vi "createMotionProfile.vi"(6 "ms per frame":dbl=50.0, 8 "Max Jerk (In/sec^3)":dbl=60.0, 9 "Max Acceleration (In/sec^2)":dbl=80.0, 10 "Max Speed (In/sec)":dbl=120.0, 11 "Inches to Travel":dbl=250.0) -> (3 "Profile":cluster{"Pos":dbl[], "Vel":dbl[], "accel":dbl[]})   [LabVIEW 2016]
panel:
  out "Final Position":dbl
  out "XY Graph":cluster{dbl[], dbl[]}[](graph)
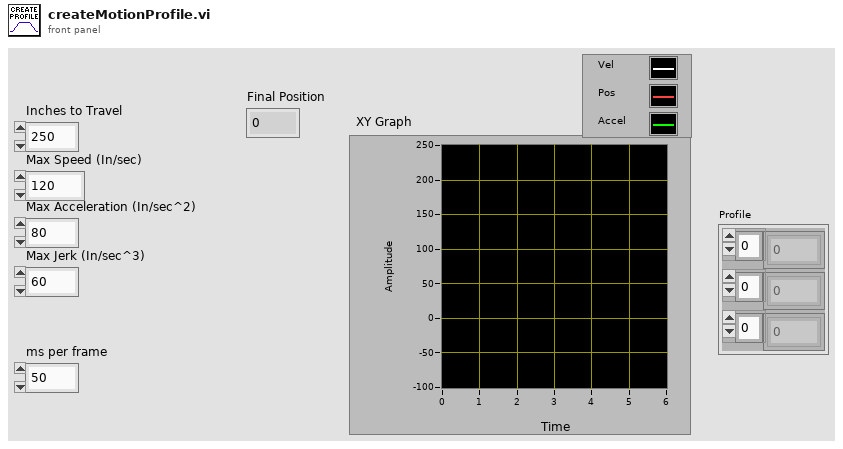
[diagram p1: front panel]
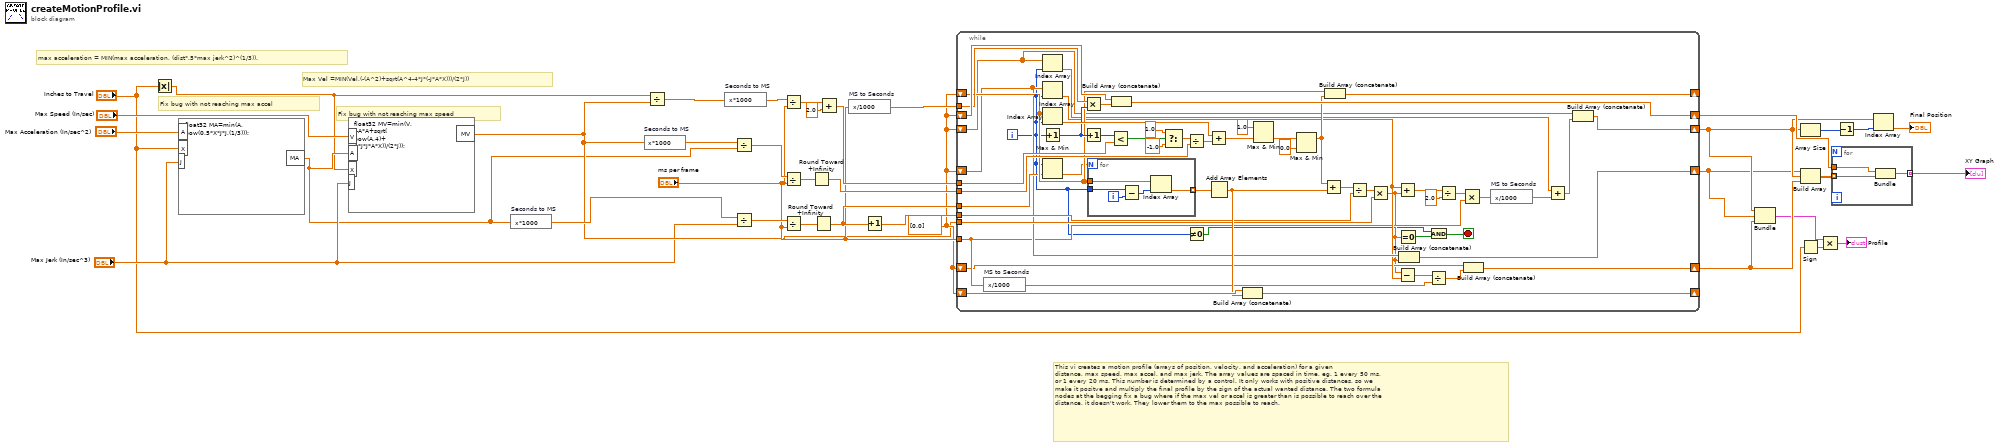
[diagram p0: block diagram]
diagram:
  w20 = dbl[] [0.0]
  # "Fix bug with not reaching max accel"
  # "max acceleration = MIN(max acceleration, (dist*.5*max jerk^2)^(1/3))."
  # "This vi creates a motion profile (arrays of position, velocity, and acceleration) for a given\ndistance, max speed, max accel, and max jerk. The array values are spaced in time, eg. 1 every 50 ms, \nor 1 every 20 ms. This number is determined by a control. It only works with positive distances, so we \nmake it positve and multiply the final profile by the sign of the actual wanted distance. The two formula\nnodes at the begging fix a bug where if the max vel or accel is greater than is possible to reach over the\ndistance, it doesn't work. They lower them to the max possible to reach."
  # "Fix bug with not reaching max speed"
  # "Max Vel =MIN(Vel,(-(A^2)+sqrt(A^4-4*J*(-J*A*X)))/(2*J))"
  n1 = Absolute Value(x="Inches to Travel") -> (abs(x)=w1:dbl)
  n2 = formula code="float32 MA=min(A,\npow(0.5*X*J*J,(1/3)));"("A"="Max Acceleration (In/sec^2)", "X"="Inches to Travel", "J"="Max Jerk (In/sec^3)") -> ("MA"=w9:sgl)
  n3 = formula code="float32 MV=min(V,\n(-A*A+sqrt(\npow(A,4)+\n4*J*J*A*X))/(2*J));"("V"="Max Speed (In/sec)", "A"=w9, "X"=w1, "J"="Max Jerk (In/sec^3)") -> ("MV"=w13:sgl)
  n4 = expression code="x*1000" "Seconds to MS"(w9) -> (w35:sgl)
  n5 = expression code="x*1000" "Seconds to MS"(w13) -> (w34:sgl)
  n6 = Divide(x=w1, y=w13) -> (x/y=w33:dbl)
  n7 = expression code="x*1000" "Seconds to MS"(w33) -> (w32:dbl)
  n8 = Divide(x=w34, y=w9) -> (x/y=w28:sgl)
  n9 = Divide(x=w35, y="Max Jerk (In/sec^3)") -> (x/y=w25:dbl)
  n10 = Divide(x=w32, y="ms per frame") -> (x/y=w31:dbl)
  n11 = Divide(x=w28, y="ms per frame") -> (x/y=w27:dbl)
  n12 = Divide(x=w25, y="ms per frame") -> (x/y=w24:dbl)
  n13 = Round Toward +Infinity(x=w27) -> (ceil(x): smallest int >= x=w26:dbl)
  n14 = Round Toward +Infinity(x=w24) -> (ceil(x): smallest int >= x=w23:dbl)
  n15 = Add(x=w31, y=2.0) -> (x+y=w29:dbl)
  n16 = expression code="x/1000" "MS to Seconds"("ms per frame") -> (w36:dbl)
  n17 = Increment(x=w23) -> (x+1=w22:dbl)
  n18 = while {
    shift-right: [w89] -> w18
    shift-left: w20 -> [w90]
    tunnel: w36 -> [w88]
    tunnel: w29 -> [w86]
    shift-right: [w72] -> _
    shift-left: w20 -> [w71]
    tunnel: w26 -> [w78]
    tunnel: w23 -> [w69]
    shift-right: [w66] -> _
    shift-left: w20 -> [w67]
    tunnel: w22 -> [w62]
    tunnel: w13 -> [w60]
    shift-right: [w59] -> w6
    shift-left: w20 -> [w57]
    shift-right: [w58] -> w8
    shift-left: w20 -> [w51]
    tunnel: "ms per frame" -> [w45]
    shift-right: [w43] -> w7
    shift-left: w20 -> [w42]
    i -> [w41]
    stop <- w37 stop-if-true
    n19 = expression code="x/1000" "MS to Seconds"(w45) -> (w46:dbl)
    n20 = Index Array(array=w51, index=w41) -> (element=w50:dbl)
    n21 = Index Array(array=w57, index=w41) -> (element=w48:dbl)
    n22 = Index Array(array=w71, index=w41) -> (element=w76:dbl)
    n23 = Increment(x=w41) -> (x+1=w74:i32)
    n24 = Max & Min(x=w41, y=w69) -> (min(x,y)=w68:dbl)  [unwired: 1 out]
    n25 = Multiply(x=w88, y=w74) -> (x*y=w87:dbl)
    n26 = Increment(x=w74) -> (x+1=w75:i32)
    n27 = for {
      N: w68 -> [_]
      tunnel: w41 -> [w94]
      tunnel: w71 -> [w92]
      tunnel: [w91] -> w70 mode=indexing
      i -> [w95]
      n28 = Subtract(x=w94, y=w95) -> (x-y=w93:i32)
      n29 = Index Array(array=w92, index=w93) -> (element=w91:dbl)
    }
    n30 = Less?(x=w75, y=w86) -> (x < y?=w82:bool)
    n31 = Build Array (concatenate)(w90, w87) -> (w89:dbl[])
    n32 = Select(t=1.0, s=w82, f=-1.0) -> (s? t:f=w79:dbl)
    n33 = Divide(x=w79, y=w78) -> (x/y=w77:dbl)
    n34 = Not Equal To 0?(x=w41) -> (x != 0?=w38:bool)
    n35 = Add(x=w76, y=w77) -> (x+y=w73:dbl)
    n36 = Add Array Elements(numeric array=w70) -> (sum=w65:dbl)
    n37 = Build Array (concatenate)(w67, w65) -> (w66:dbl[])
    n38 = Max & Min(x=1.0, y=w73) -> (min(x,y)=w84:dbl)  [unwired: 1 out]
    n39 = Max & Min(x=w84, y=0.0) -> (max(x,y)=w64:dbl)  [unwired: 1 out]
    n40 = Add(x=w64, y=w65) -> (x+y=w63:dbl)
    n41 = Build Array (concatenate)(w71, w64) -> (w72:dbl[])
    n42 = Divide(x=w63, y=w62) -> (x/y=w61:dbl)
    n43 = Multiply(x=w61, y=w60) -> (x*y=w40:dbl)
    n44 = Add(x=w48, y=w40) -> (x+y=w56:dbl)
    n45 = Subtract(x=w40, y=w48) -> (x-y=w47:dbl)
    n46 = Equal To 0?(x=w40) -> (x = 0?=w39:bool)
    n47 = Build Array (concatenate)(w57, w40) -> (w59:dbl[])
    n48 = Divide(x=w47, y=w46) -> (x/y=w44:dbl)
    n49 = And(x=w38, y=w39) -> (x .and. y?=w37:bool)
    n50 = Divide(x=w56, y=2.0) -> (x/y=w54:dbl)
    n51 = Multiply(x=w54, y=w45) -> (x*y=w53:dbl)
    n52 = Build Array (concatenate)(w42, w44) -> (w43:dbl[])
    n53 = expression code="x/1000" "MS to Seconds"(w53) -> (w52:dbl)
    n54 = Add(x=w50, y=w52) -> (x+y=w49:dbl)
    n55 = Build Array (concatenate)(w51, w49) -> (w58:dbl[])
  }
  n56 = Bundle(w8, w6, w7) -> (w5:cluster{dbl[], dbl[], dbl[]})  [unwired: 1 in]
  n57 = Array Size(array=w8) -> (size(s)=w16:i32)
  n58 = Build Array(w6, w8, w7) -> (w19:dbl[][])
  n59 = Sign(1:"Inches to Travel") -> (0:w3:dbl)
  n60 = Multiply(x=w5, y=w3) -> (x*y=→"Profile":cluster{dbl[], dbl[], dbl[]})
  n61 = for {
    tunnel: w19 -> [w98] mode=indexing
    tunnel: w18 -> [w97]
    tunnel: [w96] -> w17 mode=indexing
    n62 = Bundle(w97, w98) -> (w96:cluster{dbl[], dbl[]})  [unwired: 1 in]
  }
  "XY Graph" <- w17
  n63 = Decrement(x=w16) -> (x-1=w15:i32)
  n64 = Index Array(array=w8, index=w15) -> (element=→"Final Position":dbl)
